vi "Calculate Measurement Parameters.vi"(8 "error in":errorcluster, 9 "scaled signal in [EU]":waveform(dbl)={"t0"=timestamp(0 s since 1904-01-01), "dt"=0.0, "Y"=[]}, 10 "Full scale range":dbl, 11 "Maximum harmonic":i32) -> (0 "error out":errorcluster, 3 "Meas results":T1)   [LabVIEW 2021, in "Frequency Response_Audio ADC.lvlib"]
uses:
  Frequency Response_Audio ADC.lvlib
  <vilib>/addons/_NISVFA/_Shared subVIs/Common/SVL Set dB Reference (1 Ch).vi
  <vilib>/addons/Sound and Vibration/svt_Level/SVL AC & DC Level (Time) (1 Ch).vi
  <vilib>/addons/_NISVFA/_Shared subVIs/Controls/svc_Window.ctl
  <vilib>/addons/Sound and Vibration/svt_Distortion/SoundVib_Distortion.lvlib
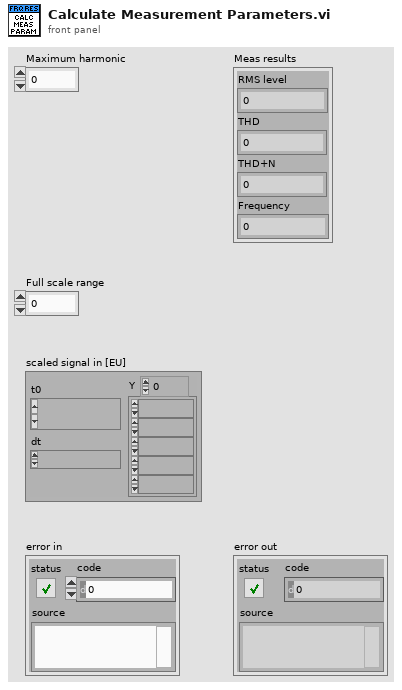
[diagram p1: front panel]
types:
  T1 = cluster{"RMS level":dbl, "THD":dbl, "THD+N":dbl, "Frequency":dbl}
  T2 = cluster{"start frequency":dbl, "stop frequency":dbl}
  T3 = cluster{"THD units":enum16{"dB", "linear ratio", "%"}, "harmonic component amplitude units":enum16{"EU rms", "EU peak", "EU peak-peak", "dB ref fund"}, "detected fundamental amplitude units":enum16{"EU rms", "EU peak", "EU peak-peak"}}
  T4 = typedef "svc_Window.ctl" = u32
  T5 = typedef "svc_Spectrum Info.ctl" = cluster{"channel name":string, "description":string, "x-axis units":T6, "spectral info":cluster{"spectrum type":T7, "linear/dB":enum16{"linear", "dB"}, "window":u16, "window size":i32, "FFT size":i32}, "engineering units":T8, "custom label":string, "dB reference [EU]":dbl, "peak units":enum16{"rms", "peak", "peak-peak"}, "weighting filter":T9, "spectral density?":bool, "unit label":string, "spectrum skewed?":bool, "complimentary spectrum units":T10}
  T6 = typedef "svc_X-Axis Units.ctl" = u16
  T7 = typedef "svc_Spectrum Type.ctl" = enum16{"FFT Spectrum [complex]", "Amplitude [Magnitude]", "Power [Magnitude^2]", "Cross Spectrum [complex]", "Frequency Response [Complex]"}
  T8 = typedef "svc_Engineering Units Text Ring.ctl" = u16
  T9 = typedef "svc_Weighting Filter Text Ring.ctl" = u16
  T10 = typedef "svc_Complimentary Spectrum Units.ctl" = enum16{"none", "radians", "degrees", "cycles", "imaginary"}
  T11 = cluster{"complex spectrum response":cluster{"f0":dbl, "df":dbl, "complex spectrum":cdb[]}, "spectrum info":T5}
  T12 = cluster{"detected fundamental\namplitude":dbl, "THD":dbl, "THD+N":dbl, "detected fundamental\nfrequency [Hz]":dbl}
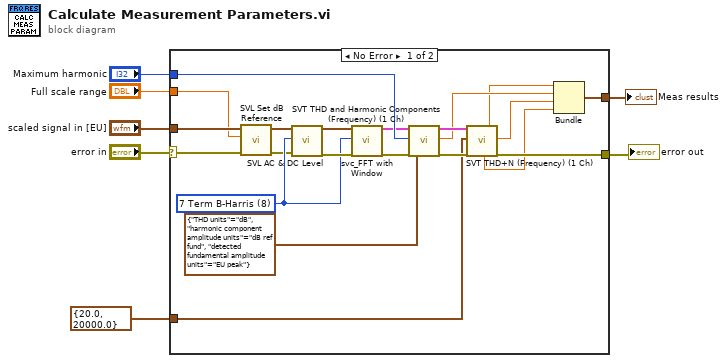
[diagram p0: block diagram]
diagram:
  n1 = case shown="No Error" "error in" {
    selector: "error in" -> [w10 w29]
    tunnel: [w28 w29] -> w7
    tunnel: "scaled signal in [EU]" -> [w27 _]
    tunnel: "Maximum harmonic" -> [w23 _]
    tunnel: "Full scale range" -> [w15 _]
    tunnel: [w11 _] -> w3
    tunnel: T2 {"start frequency"=20.0, "stop frequency"=20000.0} ("frequency range") -> [w9 _]
    frame No Error {
      w19 = T4 8 items=["None"=0, "Hanning"=1, "Hamming"=2, "Blackman-Harris"=3, "Exact Blackman"=4, "Blackman"=5, "Flat Top"=6, "4 Term B-Harris "=7, "7 Term B-Harris"=8, "Low Sidelobe"=9, "Force"=64, "Exponential"=65, "Blackman Nuttall"=11, "Triangle"=30, "Bartlett-Hanning"=31, "Bohman"=32, "Parzen"=33, "Welch"=34, "Kaiser"=60, "Dolph-Chebyshev"=61, "Gaussian"=62] ("window")
      n2 = call-poly <vilib>:"SVL Set dB Reference.vi"("error in (no error)"=w10, "dB reference [EU]"=w15, "scaled signal in [EU]"=w27) -> ("error out"=w17:errorcluster, "scaled signal out [EU]"=w16:waveform(dbl))  [unwired: 7 in]
      n3 = call-poly <vilib>:"SVL AC & DC Level.vi"("scaled signal [EU]"=w16, "window"=w19, "error in (no error)"=w17) -> ("AC signal [EU]"=w18:waveform(dbl), "error out"=w20:errorcluster)  [unwired: 11 in, 4 out]
      n4 = call <vilib>:"svc_FFT with Window.vi"("time signal in [EU]"=w18, "window"=w19, "error in"=w20) -> ("complex spectrum"=w22:T11, "error out"=w21:errorcluster)  [unwired: 15 in]
      n5 = call <vilib>:"SVT THD and Harmonic Components (Frequency) (1 Ch).vi"("complex spectrum"=w22, "maximum harmonic"=w23, "error in (no error)"=w21, "desired units"=T3 {"THD units"=enum."dB", "harmonic component amplitude units"=enum."dB ref fund", "detected fundamental amplitude units"=enum."EU peak"}) -> ("complex spectrum"=w26:T11, "THD"=w14:dbl, "error out"=w25:errorcluster)  [unwired: 8 in, 5 out]
      n6 = call <vilib>:"SVT THD+N (Frequency) (1 Ch).vi"("complex spectrum"=w26, "frequency range"=w9, "error in (no error)"=w25) -> ("detected fundamental\nfrequency [Hz]"=w12:dbl, "detected fundamental\namplitude"=w8:dbl, "THD+N"=w13:dbl, "error out"=w28:errorcluster)  [unwired: 11 in, 2 out]
      n7 = Bundle("detected fundamental\namplitude"=w8, "THD"=w14, "THD+N"=w13, "detected fundamental\nfrequency [Hz]"=w12) -> (w11:T12)  [unwired: 1 in]
    }
    frame Error {
    }
  }
  "error out" <- w7
  "Meas results" <- w3
